vi "is exe.vi"() -> (1 "Path":path)   [LabVIEW 2017]
panel:
  out "path":path
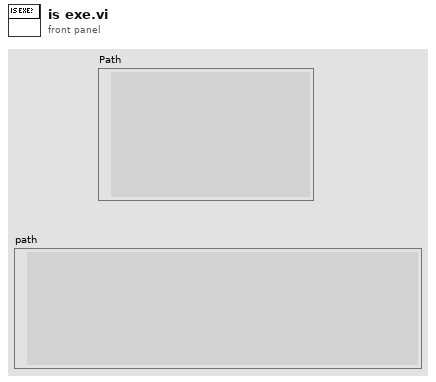
[diagram p1: front panel]
types:
  T1 = enum32{"invalid app kind", "Development System", "Run Time System", "Student Edition", "Embedded LabVIEW", "Evaluation", "Custom"}
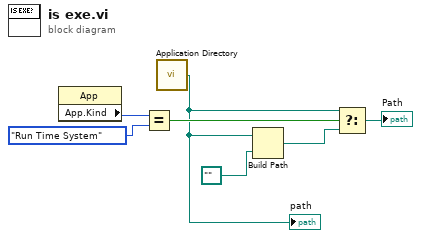
[diagram p0: block diagram]
diagram:
  n1 = property class="App"() -> ("App.Kind"=w7:T1)  [unwired: 2 in, 2 out]
  n2 = Equal?(x=w7, y=T1."Run Time System") -> (x = y?=w5:bool)
  n3 = call <vilib>:"Application Directory.vi"() -> ("Application Directory"=w1:path)
  "path" <- w1
  n4 = Build Path(base path=w1, name or relative path=path ".." ("path")) -> (appended path=w3:path)
  n5 = Select(t=w1, s=w5, f=w3) -> (s? t:f=→"Path":path)
